vi "Get Transfer Group by ID.vi"(10 "Transfer Group id":i32, 11 "Cache in":refnum<class "Memory Cache.lvclass">) -> (2 "Transfer Group":refnum<class "DSF.Engine.Transfer Group.lvclass">, 3 "Cache out":refnum<class "Memory Cache.lvclass">)   [LabVIEW 2017, in "Data Sharing Framework Engine.lvlib" / "Memory Cache.lvclass"]
uses:
  Memory Cache.lvclass
  old/dsf core/Source/Engine/Classes/Transfer/DSF.Engine.Transfer Group.lvclass
  Memory Cache.lvclass/Memory Cache.ctl
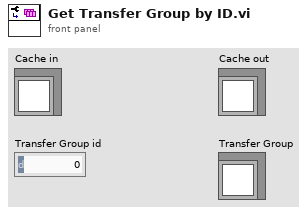
[diagram p1: front panel]
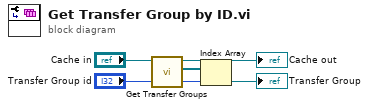
[diagram p0: block diagram]
diagram:
  n1 = call "Get Transfer Groups.vi"("Cache in"="Cache in") -> ("Transfers Groups"=w3:refnum<class "DSF.Engine.Transfer Group.lvclass">[], "Cache out"=→"Cache out":refnum<class "Memory Cache.lvclass">)  [unwired: 9 in]
  n2 = Index Array(array=w3, index="Transfer Group id") -> (element=→"Transfer Group":refnum<class "DSF.Engine.Transfer Group.lvclass">)
